vi "IK.vi"(8 "Underhand?":bool, 9 "Collector X Position [m]":dbl, 10 "Collector Z Position [m]":dbl, 11 "Robot Dimensions":T1) -> (1 "2nd Joint Angle":dbl, 2 "1st Joint Angle":dbl)   [LabVIEW 2011]
panel:
  out "2nd Joint Degrees":dbl
  out "1st Joint Degrees":dbl
  # "2nd joint angle"
  # "2nd joint"
  # "1st joint angle"
  # "1st joint"
  # "z"
  # "x"
  # "z-offset"
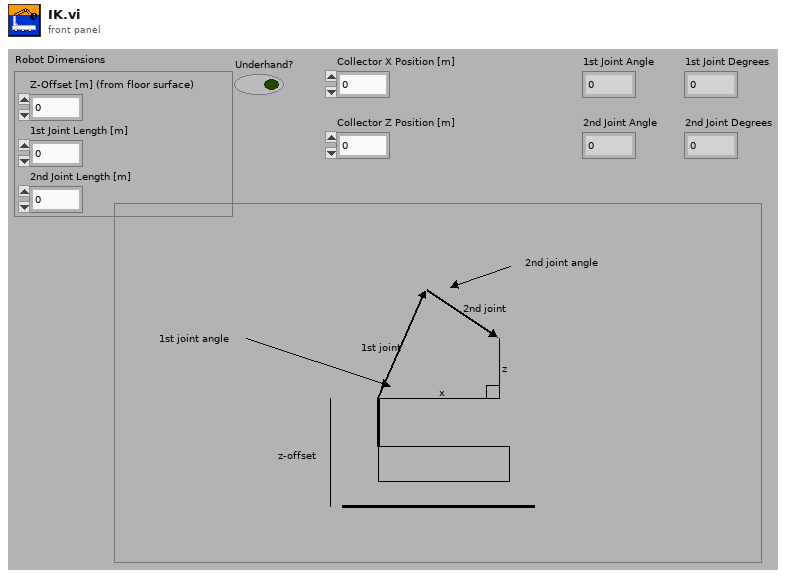
[diagram p1: front panel]
types:
  T1 = cluster{"Z-Offset [m] (from floor surface)":dbl, "1st Joint Length [m]":dbl, "2nd Joint Length [m]":dbl}
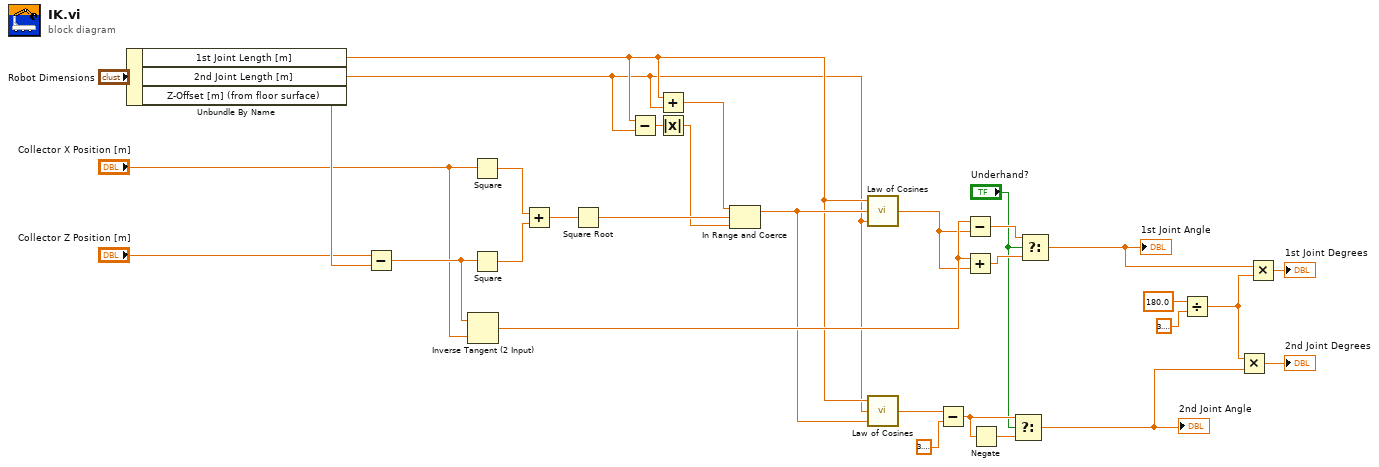
[diagram p0: block diagram]
diagram:
  n1 = Unbundle By Name("Robot Dimensions") -> ("1st Joint Length [m]"=w5:dbl, "2nd Joint Length [m]"=w4:dbl, "Z-Offset [m] (from floor surface)"=w27:dbl)
  n2 = Subtract(x="Collector Z Position [m]", y=w27) -> (x-y=w28:dbl)
  n3 = Inverse Tangent (2 Input)(1:"Collector X Position [m]", 2:w28) -> (0:w18:dbl)
  n4 = Square(x="Collector X Position [m]") -> (x^2=w30:dbl)
  n5 = Square(x=w28) -> (x^2=w29:dbl)
  n6 = Add(x=w30, y=w29) -> (x+y=w26:dbl)
  n7 = Square Root(x=w26) -> (sqrt(x)=w6:dbl)
  n8 = Subtract(x=w5, y=w4) -> (x-y=w3:dbl)
  n9 = Add(x=w5, y=w4) -> (x+y=w2:dbl)
  n10 = Absolute Value(x=w3) -> (abs(x)=w1:dbl)
  n11 = In Range and Coerce(upper limit=w2, x=w6, lower limit=w1) -> (coerced(x)=w7:dbl)  [unwired: 1 out]
  n12 = call "Law of Cosines.vi"("c"=w4, "b"=w7, "a"=w5) -> ("Gamma"=w17:dbl)
  n13 = call "Law of Cosines.vi"("c"=w7, "b"=w4, "a"=w5) -> ("Gamma"=w13:dbl)
  n14 = Subtract(x=w13, y=3.141592653589793) -> (x-y=w10:dbl)
  n15 = Subtract(x=w18, y=w17) -> (x-y=w15:dbl)
  n16 = Add(x=w18, y=w17) -> (x+y=w16:dbl)
  n17 = Negate(x=w10) -> (-x=w11:dbl)
  n18 = Select(t=w10, s="Underhand?", f=w11) -> (s? t:f=w8:dbl)
  "2nd Joint Angle" <- w8
  n19 = Select(t=w15, s="Underhand?", f=w16) -> (s? t:f=w14:dbl)
  "1st Joint Angle" <- w14
  n20 = Divide(x=180.0, y=3.141592653589793) -> (x/y=w22:dbl)
  n21 = Multiply(x=w22, y=w8) -> (x*y=→"2nd Joint Degrees":dbl)
  n22 = Multiply(x=w14, y=w22) -> (x*y=→"1st Joint Degrees":dbl)
